vi "Init_Instr.vi"(8 "error in (no error)":errorcluster caption="entrée d'erreur (pas d'erreur)", 11 "Class Instrument Power_Supply en entrée":refnum<class "Class Instrument Power_Supply.lvclass">) -> (0 "error out":errorcluster caption="sortie d'erreur", 3 "Class Instrument Power_Supply en sortie":refnum<class "Class Instrument Power_Supply.lvclass">)   [LabVIEW 2020, in "Library Instrument & Equipement.lvlib" / "Library Instruments.lvlib" / "Class Instrument Power_Supply.lvclass"]
uses:
  Class Instrument Power_Supply.lvclass
  Class Instrument Power_Supply.lvclass/Class Instrument Power_Supply.ctl
  Instrument (Default)/Class Instrument (Default).lvclass
  Power_Supply/Power_Supply (Default)/Power_Supply (Default).lvclass
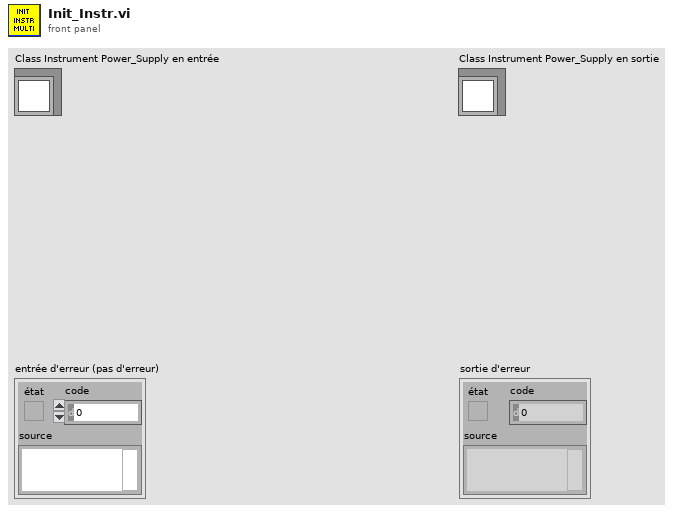
[diagram p1: front panel]
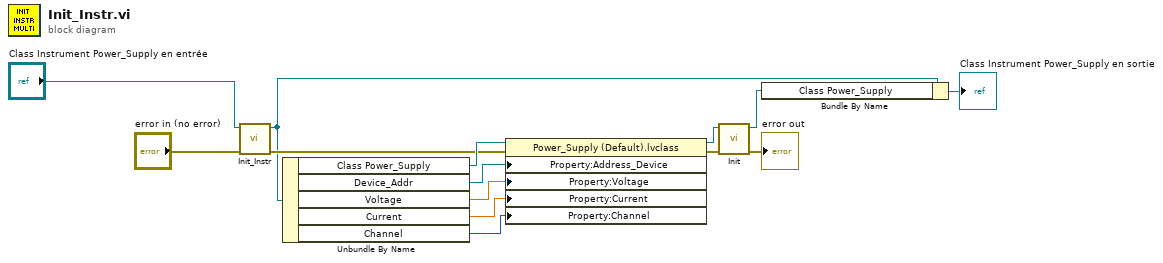
[diagram p0: block diagram]
diagram:
  n1 = call-parent "Init_Instr.vi"("error in (no error)"="error in (no error)", "Class Instrument (Default) en entrée"="Class Instrument Power_Supply en entrée") -> ("error out"=w7:errorcluster, "Class Instrument (Default) en sortie"=w4:refnum<class "Class Instrument Power_Supply.lvclass">)  [unwired: 8 in]
  n2 = Unbundle By Name(w4) -> ("Class Power_Supply"=w12:refnum<class "Power_Supply (Default).lvclass">, "Device_Addr"=w11:refnum<visa-resource-name>, "Voltage"=w10:dbl, "Current"=w9:dbl, "Channel"=w8:i32)
  n3 = property class="Power_Supply (Default).lvclass"(reference=w12, error in=w7, "Property:Address_Device"=w11, "Property:Voltage"=w10, "Property:Current"=w9, "Property:Channel"=w8) -> (reference out=w2:refnum<class "Power_Supply (Default).lvclass">, error out=w6:errorcluster)
  n4 = call-dynamic "Init.vi"("error in (no error)"=w6, "Power_Supply (Default) en entrée"=w2) -> ("error out"=→"error out":errorcluster, "Power_Supply (Default) en sortie"=w1:refnum<class "Power_Supply (Default).lvclass">)  [unwired: 8 in]
  n5 = Bundle By Name(cluster=w4, "Class Power_Supply"=w1) -> (→"Class Instrument Power_Supply en sortie":refnum<class "Class Instrument Power_Supply.lvclass">)
